vi "Set Trailing Slash.vi"(7 "Trailing Slash":bool, 11 "Path In":string) -> (3 "Path":string)   [LabVIEW 2020, in "Stream.lvlib"]
uses:
  Stream.lvlib
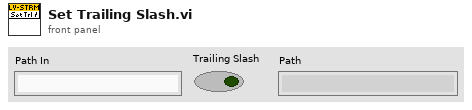
[diagram p1: front panel]
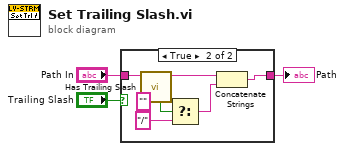
[diagram p0: block diagram]
diagram:
  n1 = case shown="True" "Trailing Slash" {
    tunnel: "Path In" -> [w4 w11]
    tunnel: [w4 w5] -> w2
    frame False {
    }
    frame True {
      n2 = call "Has Trailing Slash.vi"("Path In"=w11) -> ("Path"=w7:string, "Trailing Slash?"=w10:bool)  [unwired: 9 in]
      n3 = Select(t="", s=w10, f="/") -> (s? t:f=w6:string)
      n4 = Concatenate Strings(w7, w6) -> (w5:string)
    }
  }
  "Path" <- w2
